vi "FTW-Test-dotNET-SQLFetch.vi"() -> (0 "Test Result":errorcluster)   [LabVIEW 2015]
uses:
  System.Data
  src/time/FTW-Time-RelativeTimer.vi
  src/error/FTW-ERR-Assert-DeveloperError.vi
  src/error/FTW-ERR-ThrowError.vi
  src/error/FTW-ERR-ThrowInfo.vi
  src/error/FTW-ERR-CallChain.vi
  src/string/FTW-STR-ReplaceWhitespace.vi
  src/string/FTW-STR-Array-Delimit.vi
  src/error/FTW-ERR-Clear.vi
  src/regex/FTW-Regex-ReplaceAll.vi
  codegen/xnode/FTW-dotNet-SQL-Fetch.xnode
panel:
  out "Tables in Database":cluster{"table_name":string}[](array[cluster])
  out "ServerVersion":string
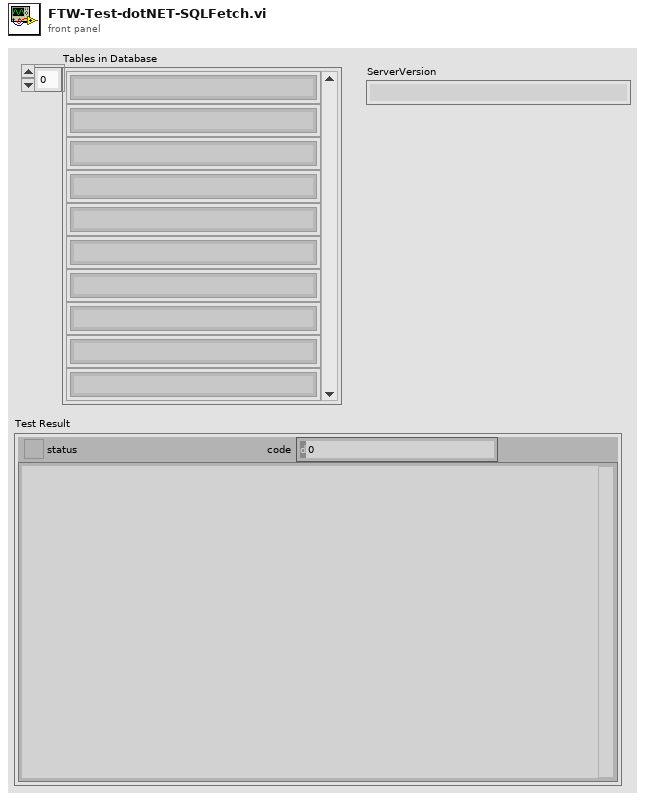
[diagram p1: front panel]
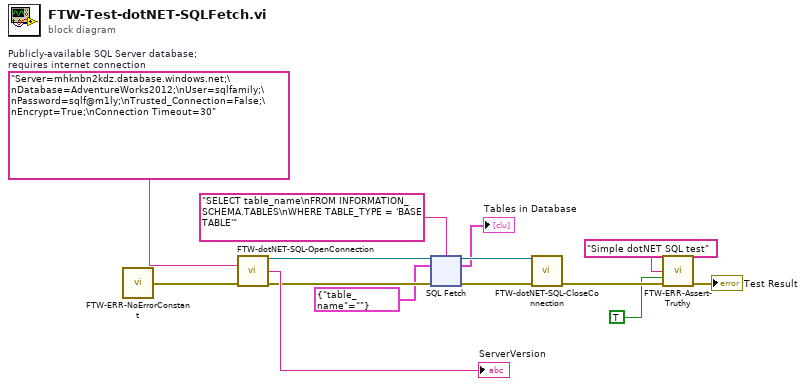
[diagram p0: block diagram]
diagram:
  w8 = "Server=mhknbn2kdz.database.windows.net;\nDatabase=AdventureWorks2012;\nUser=sqlfamily;\nPassword=sqlf@m1ly;\nTrusted_Connection=False;\nEncrypt=True;\nConnection Timeout=30"  # Publicly-available SQL Server database; requires internet connection
  n1 = call "FTW-ERR-NoErrorConstant.vi"() -> ("no error"=w12:errorcluster)
  n2 = call "FTW-dotNET-SQL-OpenConnection.vi"("Connection String"=w8, "error in"=w12) -> ("DB Connection"=w3:refnum<k24>, "ServerVersion"=→"ServerVersion":string, "error out"=w5:errorcluster)  [unwired: 11 in]
  n3 = xnode "SQL Fetch"("Connection"=w3, "SQL Script"="SELECT table_name\nFROM INFORMATION_SCHEMA.TABLES\nWHERE TABLE_TYPE = 'BASE TABLE'", "Row Datatype"=cluster{"table_name":string} {"table_name"=""}, "error in"=w5) -> ("Connection out"=w7:refnum<k24>, "Result Set"=→"Tables in Database":cluster{"table_name":string}[], "error out"=w4:errorcluster)  [unwired: 1 out]
  n4 = call "FTW-dotNET-SQL-CloseConnection.vi"("DB Connection"=w7, "error in"=w4) -> ("error out"=w10:errorcluster)  [unwired: 13 in]
  n5 = call "FTW-ERR-Assert-Truthy.vi"("Assertion"="Simple dotNET SQL test", "Assertion holds true?"=TRUE, "error in"=w10) -> ("error out"=→"Test Result":errorcluster)  [unwired: 12 in]
